vi "BP FilterI16.vi"(2 "sample rate MHz":u16, 4 "Filter Prams":T1={"Filter"=FALSE, "low cutoff"=5, "order"=81, "high cutoff"=35}, 5 "filter type":T2(ring)=enum."Bandpass", 6 "Array in":i16[][](array[numeric])) -> (0 "Filtered X":dbl[][](array[numeric]))   [LabVIEW 2022 SP3]
uses:
  <vilib>/Analysis/4window.llb/windowTd.ctl
  <vilib>/Analysis/2dsp.llb/1D Convolution (DBL).vi
  <vilib>/Analysis/3filter.llb/Chebyshev Filter (DBL).vi
  <vilib>/Analysis/NI_AALPro.lvlib
  <vilib>/Analysis/NI_AALBase.lvlib
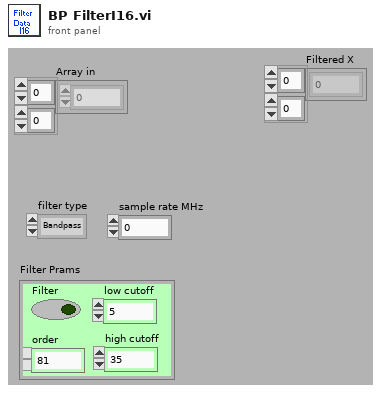
[diagram p1: front panel]
types:
  T1 = cluster{"Filter":bool, "low cutoff":i32, "order":i32, "high cutoff":i32}
  T2 = enum32{"Lowpass", "Highpass", "Bandpass", "Bandstop"}
  T3 = typedef "NI_AALPro.lvlib/windowTd.ctl" = u32
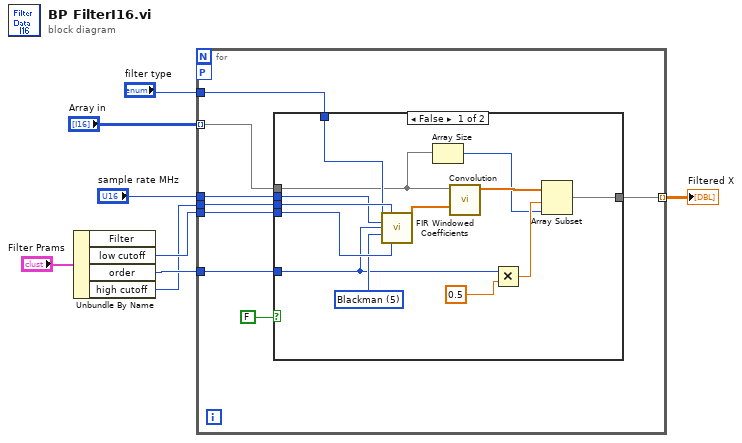
[diagram p0: block diagram]
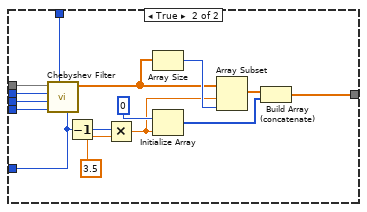
[diagram p2: hidden frame]
diagram:
  n1 = Unbundle By Name("Filter Prams") -> ("low cutoff"=w4:i32, "order"=w5:i32, "high cutoff"=w3:i32)  [unwired: 1 out]
  n2 = for {
    tunnel: "sample rate MHz" -> [w16]
    tunnel: w4 -> [w15]
    tunnel: w3 -> [w14]
    tunnel: w5 -> [w13]
    tunnel: "filter type" -> [w12]
    tunnel: [w10] -> w1 mode=indexing
    tunnel: "Array in" -> [w9] mode=indexing
    workers-P: _ -> [_]
    n3 = case shown="False" FALSE ("Case Constant\n(See Context Help)") {
      tunnel: w16 -> [w27 w44]
      tunnel: w15 -> [w23 w43]
      tunnel: w14 -> [w28 w42]
      tunnel: w9 -> [w19 w35]
      tunnel: [w24 w33] -> w10
      tunnel: w13 -> [w20 w32]
      tunnel: w12 -> [w26 w30]
      frame False {
        w21 = T3 5 items=["Rectangle"=0, "Hanning"=1, "Hamming"=2, "Blackman-Harris"=3, "Exact Blackman"=4, "Blackman"=5, "Flat Top"=6, "4 Term B-Harris "=7, "7 Term B-Harris"=8, "Low Sidelobe"=9, "Blackman Nuttall"=11, "Triangle"=30, "Bartlett-Hanning"=31, "Bohman"=32, "Parzen"=33, "Welch"=34, "Kaiser"=60, "Dolph-Chebyshev"=61, "Gaussian"=62] ("window")
        n4 = call <vilib>:"FIR Windowed Coefficients.vi"("filter type"=w26, "high cutoff freq: fh"=w28, "sampling freq: fs"=w27, "taps"=w20, "window"=w21, "low cutoff freq: fl"=w23) -> ("FIR Windowed Coefficients"=w29:dbl[])  [unwired: 2 in, 7 out]
        n5 = Array Size(array=w19) -> (size(s)=w17:i32)
        n6 = call-poly <vilib>:"Convolution.vi"("Y"=w29, "X"=w19) -> ("X * Y"=w25:dbl[])  [unwired: 1 in, 8 out]
        n7 = Multiply(x=w20, y=0.5) -> (x*y=w18:dbl)
        n8 = Array Subset(array=w25, index=w18, length=w17) -> (w24:dbl[])
      }
      frame True {
        n9 = call-poly <vilib>:"Chebyshev Filter.vi"("order"=w32, "filter type"=w30, "low cutoff freq: fl"=w43, "high cutoff freq: fh"=w42, "sampling freq: fs"=w44, "X"=w35) -> ("Filtered X"=w34:dbl[])  [unwired: 2 in, 3 out]
        n10 = Decrement(x=w32) -> (x-1=w31:i32)
        n11 = Multiply(x=w31, y=3.5) -> (x*y=w36:dbl)
        n12 = Array Size(array=w34) -> (size(s)=w39:i32)
        n13 = Initialize Array(0, w36) -> (w38:i32[])
        n14 = Array Subset(array=w34, index=w36, length=w39) -> (w37:dbl[])
        n15 = Build Array (concatenate)(w37, w38) -> (w33:dbl[])
      }
    }
  }
  "Filtered X" <- w1
